vi "Update Configuration Control.vi"(6 "Configuration reference":refnum<vi>, 8 "error in (no error)":errorcluster, 10 "Not Valid":bool, 11 "JSON Configuration":string) -> (0 "error out":errorcluster)   [LabVIEW 2021, in "CIF Template UI.lvlib"]
uses:
  CIF Template UI.lvlib
  <vilib>/addons/_JKI.lib/Serialization/JSON/JKI JSON Serialization.lvlib
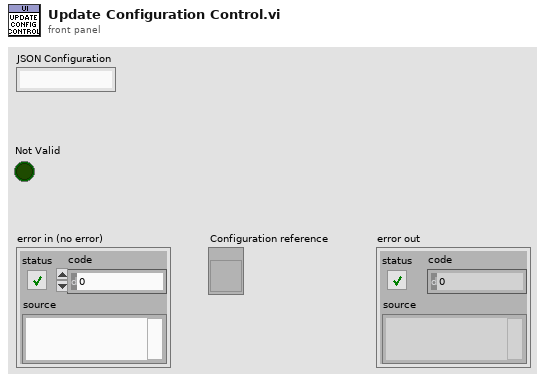
[diagram p1: front panel]
types:
  T1 = typedef "TemplateCommon.lvlib/Configuration.ctl" = cluster{"Common":T2, "Step":u64}
  T2 = typedef "CIFCoreCommon.lvlib/Common Plugin Configuration.ctl" = cluster{"Period (s)":dbl, "Offset (us)":i32, "ClockID":u8, "Priority":i32, "Processor":i32}
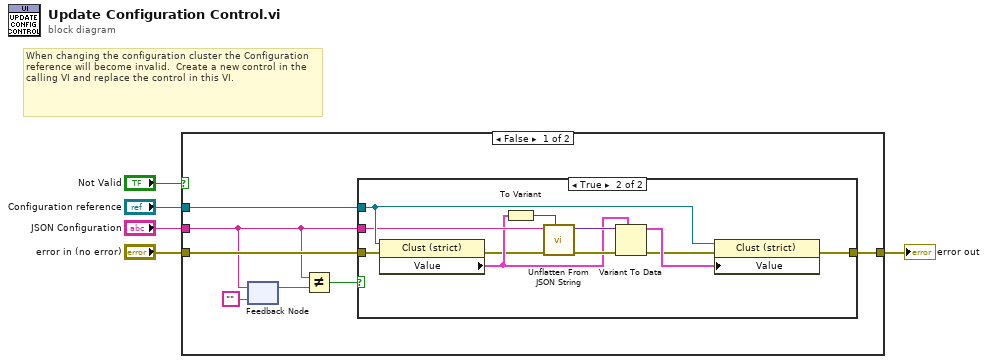
[diagram p0: block diagram]
diagram:
  # "When changing the configuration cluster the Configuration reference will become invalid.  Create a new control in the calling VI and replace the control in this VI."
  n1 = case shown="False" "Not Valid" {
    tunnel: [w12 w25] -> w1
    tunnel: "error in (no error)" -> [w11 w25]
    tunnel: "Configuration reference" -> [w10 _]
    tunnel: "JSON Configuration" -> [w8 _]
    frame False {
      n2 = feedback #1("" ("JSON Configuration")) -> (w7:string)
      n3 = feedback-in #1(w8) -> ()
      n4 = Not Equal?(x=w8, y=w7) -> (x != y?=w6:bool)
      n5 = case shown="True" w6 {
        tunnel: [w13 w24] -> w12
        tunnel: w11 -> [w13 w15]
        tunnel: w10 -> [_ w23]
        tunnel: w8 -> [_ w19]
        frame False {
        }
        frame True {
          n6 = property class="Clust (strict)"(reference=w23, error in=w15) -> (error out=w14:errorcluster, "Value"=w17:T1)  [unwired: 1 out]
          n7 = To Variant(anything=w17) -> (Variant=w16:variant)
          n8 = call <vilib>:"Unflatten From JSON String.vi"("Type and Defaults"=w16, "error in (no error)"=w14, "JSON String"=w19) -> ("error out"=w18:errorcluster, "Variant"=w22:variant)  [unwired: 7 in]
          n9 = Variant To Data(error in=w18, type=w17, Variant=w22) -> (data=w21:T1, error out=w20:errorcluster)
          n10 = property class="Clust (strict)"(reference=w23, error in=w20, "Value"=w21) -> (error out=w24:errorcluster)  [unwired: 1 out]
        }
      }
    }
    frame True {
    }
  }
  "error out" <- w1
